vi "Generate logfile path 2.vi"(8 "error in":errorcluster, 10 "Típus":string, 11 "Etalon number":u32) -> (0 "error out":errorcluster, 2 "Log_Path":path)   [LabVIEW 2014]
panel:
  out "File name":string
  out "Folder exists?":bool
  out "Folder path":path
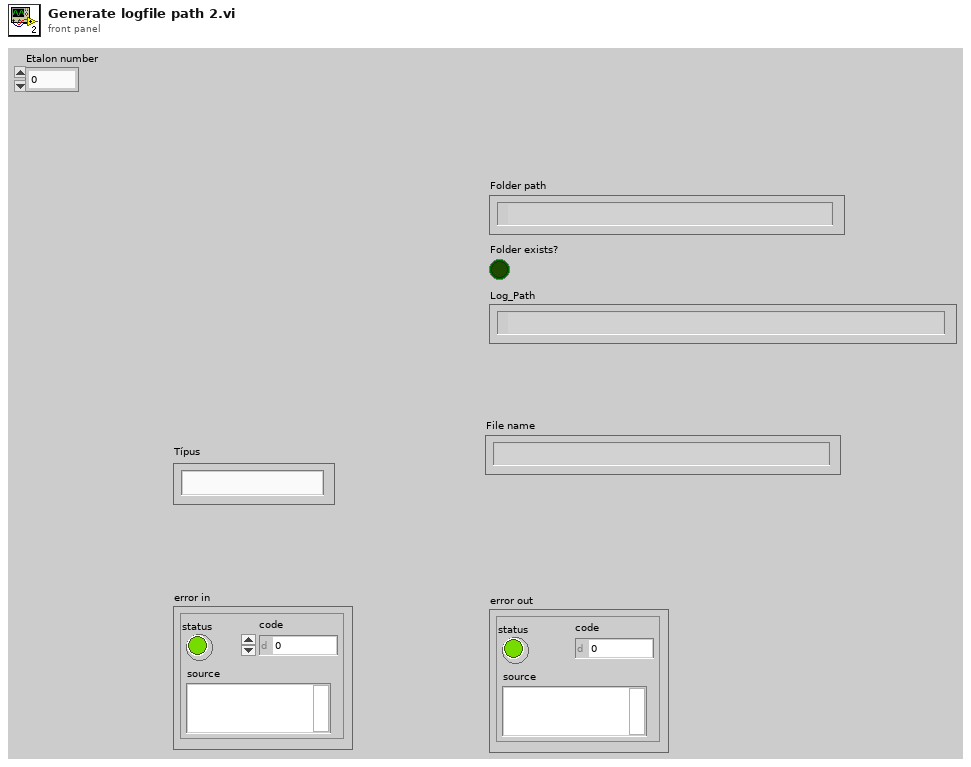
[diagram p1: front panel]
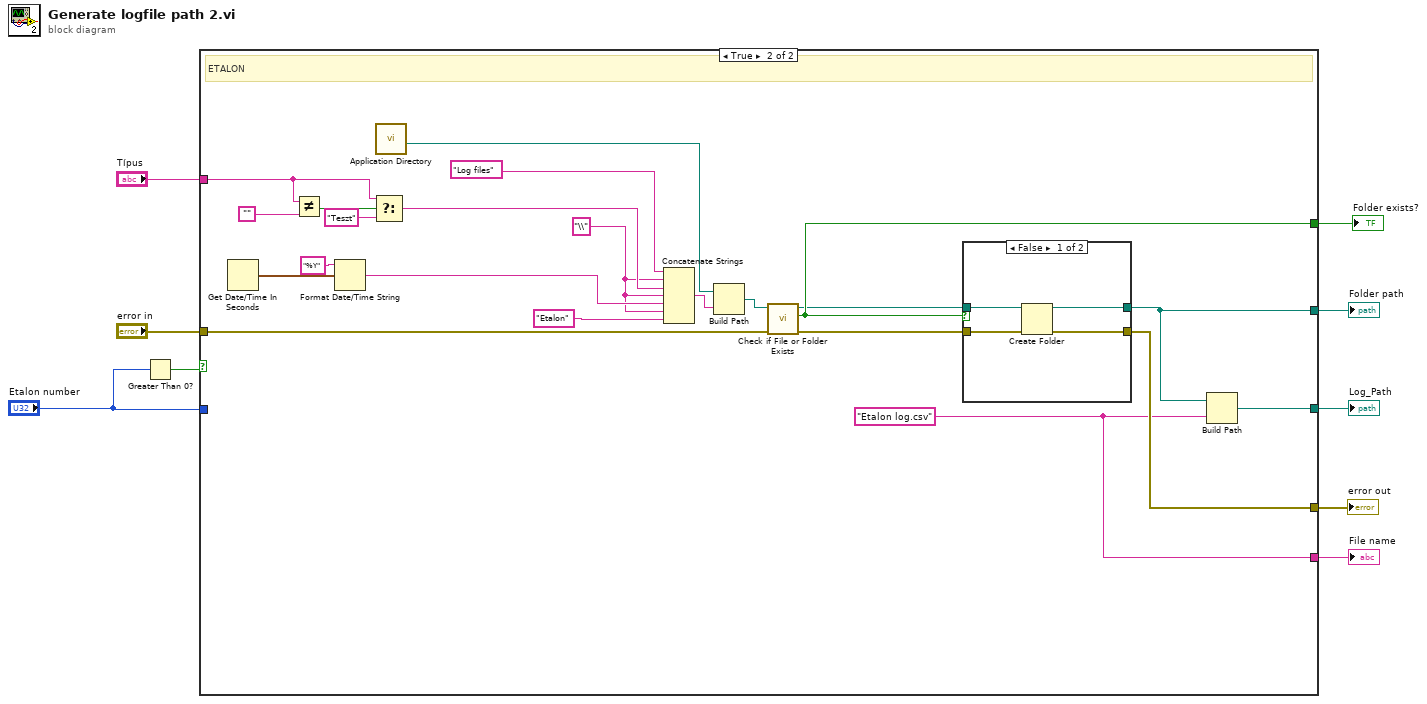
[diagram p0: block diagram]
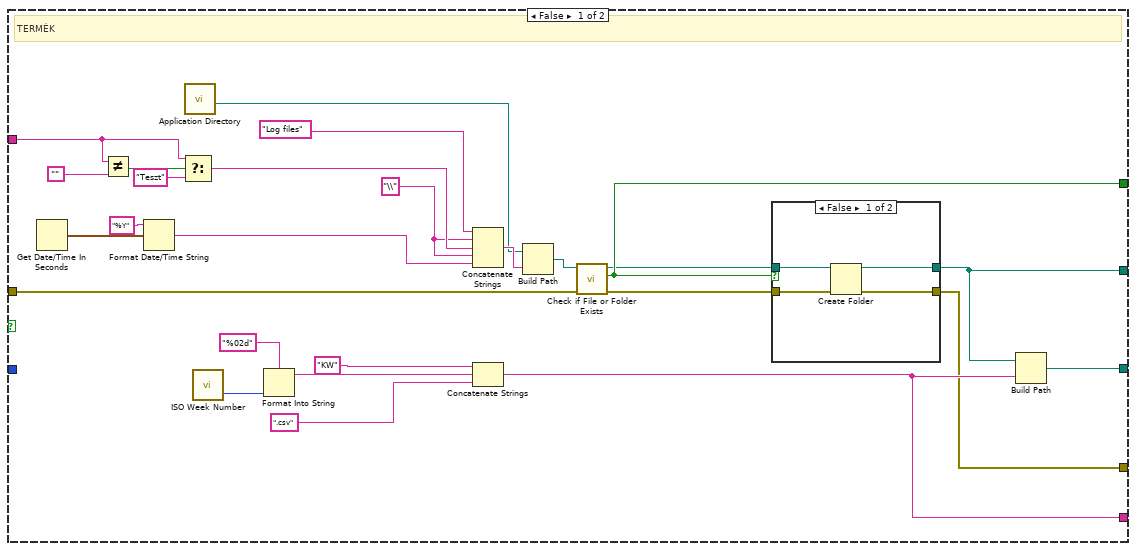
[diagram p2: hidden frame]
diagram:
  n1 = Greater Than 0?(x="Etalon number") -> (x > 0?=w2:bool)
  n2 = case shown="True" w2 {
    tunnel: "error in" -> [w35 w63]
    tunnel: [w34 w62] -> w8
    tunnel: [w33 w61] -> w7
    tunnel: [w32 w60] -> w6
    tunnel: [w31 w42] -> w5
    tunnel: [w30 w59] -> w4
    tunnel: "Típus" -> [w14 w48]
    tunnel: "Etalon number" -> [_ _]
    frame False {
      w10 = "\\" ("prompt (Choose or enter file path)")
      # "TERMÉK"
      n3 = Get Date/Time In Seconds() -> (seconds since 1Jan1904=w29:timestamp)
      n4 = Not Equal?(x=w14, y="") -> (x != y?=w15:bool)
      n5 = Format Date/Time String(time format string (%c)="%Y", seconds (now)=w29) -> (date/time string=w21:string)  [unwired: 1 in]
      n6 = Select(t=w14, s=w15, f="Teszt") -> (s? t:f=w12:string)
      n7 = call <vilib>:"Application Directory.vi"() -> ("Application Directory"=w20:path)
      n8 = call "ISO Week Number.vi"() -> ("ISO week"=w23:i32)  [unwired: 2 out]
      n9 = Format Into String(format string="%02d", w23) -> (resulting string=w18:string)  [unwired: 2 in, 1 out]
      n10 = Concatenate Strings("Log files" ("prompt (Choose or enter file path)"), w10, w12, w10, w21) -> (w27:string)
      n11 = Concatenate Strings("KW" ("string"), w18, ".csv" ("string")) -> (w31:string)
      n12 = Build Path(base path=w20, name or relative path=w27) -> (appended path=w26:path)
      n13 = call <vilib>:"Check if File or Folder Exists.vi"("error in (no error)"=w35, "path"=w26) -> ("error out"=w24:errorcluster, "file or folder exists?"=w34:bool, "dup path"=w25:path)  [unwired: 7 in]
      n14 = case shown="False" w34 {
        tunnel: w25 -> [w39 w41]
        tunnel: [w36 w41] -> w33
        tunnel: w24 -> [w38 w40]
        tunnel: [w37 w40] -> w30
        frame False {
          n15 = Create Folder(path (use dialog)=w39, error in=w38) -> (created path=w36:path, error out=w37:errorcluster)  [unwired: 1 in, 1 out]
        }
        frame True {
        }
      }
      n16 = Build Path(base path=w33, name or relative path=w31) -> (appended path=w32:path)
    }
    frame True {
      w44 = "\\" ("prompt (Choose or enter file path)")
      w42 = "Etalon log.csv" ("string")
      # "ETALON"
      n17 = Get Date/Time In Seconds() -> (seconds since 1Jan1904=w58:timestamp)
      n18 = Not Equal?(x=w48, y="") -> (x != y?=w49:bool)
      n19 = Format Date/Time String(time format string (%c)="%Y", seconds (now)=w58) -> (date/time string=w52:string)  [unwired: 1 in]
      n20 = Select(t=w48, s=w49, f="Teszt") -> (s? t:f=w46:string)
      n21 = call <vilib>:"Application Directory.vi"() -> ("Application Directory"=w51:path)
      n22 = Concatenate Strings("Log files" ("prompt (Choose or enter file path)"), w44, w46, w44, w52, w44, "Etalon" ("f")) -> (w57:string)
      n23 = Build Path(base path=w51, name or relative path=w57) -> (appended path=w56:path)
      n24 = call <vilib>:"Check if File or Folder Exists.vi"("error in (no error)"=w63, "path"=w56) -> ("error out"=w54:errorcluster, "file or folder exists?"=w62:bool, "dup path"=w55:path)  [unwired: 7 in]
      n25 = case shown="False" w62 {
        tunnel: w55 -> [w67 w69]
        tunnel: [w64 w69] -> w61
        tunnel: w54 -> [w66 w68]
        tunnel: [w65 w68] -> w59
        frame False {
          n26 = Create Folder(path (use dialog)=w67, error in=w66) -> (created path=w64:path, error out=w65:errorcluster)  [unwired: 1 in, 1 out]
        }
        frame True {
        }
      }
      n27 = Build Path(base path=w61, name or relative path=w42) -> (appended path=w60:path)
    }
  }
  "Folder exists?" <- w8
  "Folder path" <- w7
  "Log_Path" <- w6
  "error out" <- w4
  "File name" <- w5
